vi "Complex Matrix Power.vi"(2 "n":i32, 3 "Input Matrix":T1) -> (0 "error":i32, 1 "Matrix Power":T1)   [LabVIEW 2017, in "NI_AALBase.lvlib"]
doc: "Computes the nth power of <B>Input Matrix</B>. Wire data to the <B>Input Matrix</B> input to determine the polymorphic instance to use or manually select the instance."
uses:
  <vilib>/Analysis/NI_AALBase.lvlib
  <vilib>/Analysis/Matrix/Datatypes/ComplexMatrix.ctl
  <resource>/lvanlys.dll
  <vilib>/Analysis/Matrix/NI_Matrix.lvlib
panel:
  # "Power of  Matrix"
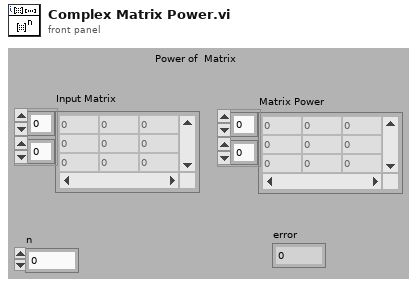
[diagram p1: front panel]
types:
  T1 = typedef "NI_Matrix.lvlib/ComplexMatrix.ctl" = cdb[][]
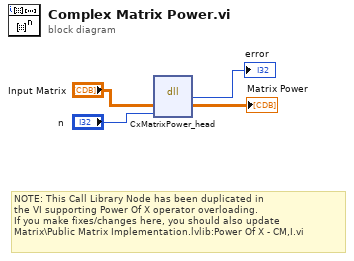
[diagram p0: block diagram]
diagram:
  # "NOTE: This Call Library Node has been duplicated in\nthe VI supporting Power Of X operator overloading.\nIf you make fixes/changes here, you should also update\nMatrix\\Public Matrix Implementation.lvlib:Power Of X - CM,I.vi"
  n1 = dll-call lib="e:/builds/penguin/labview/branches/2017/dev/dist/resource/lvanlys.*" fn="CxMatrixPower_head"("Input Matrix"="Input Matrix", "p"="n") -> (→"error":i32, "Input Matrix"=→"Matrix Power":T1)  [unwired: 4 in, 2 out]
